vi "AWG IV measurement.vi"() -> ()   [LabVIEW 2024]
uses:
  <vilib>/LabVIEW Targets/FPGA/cRIO/shared/nicrio_ModuleControls/nicrio_cRIO-9775_TriggerSlope.ctl
  <vilib>/LabVIEW Targets/FPGA/cRIO/shared/nicrio_ModuleControls/nicrio_BasicConversionTime.ctl
  <vilib>/LabVIEW Targets/FPGA/cRIO/shared/nicrio_ModuleControls/nicrio_cRIO-9775_RecordDataRates4ChansRing.ctl
  Ramps.ctl
  <vilib>/rvi/Emulation/niFpgaGetClockAttributes.vi
  <vilib>/rvi/Emulation/niFpgaSctlEmulationGetInTimedLoop.vi
  <vilib>/rvi/Emulation/niFpgaEmulationReportErrorSimple.vi
  <vilib>/rvi/eio/common/nirviEmuTemplateMethod_errors.vi
  <vilib>/rvi/Emulation/niFpgaCriticalErrorInLSC.vi
  <vilib>/rvi/Emulation/niFpgaProcessEmulError.vi
  <vilib>/rvi/Emulation/niFpgaEmulationIsFPGAContextNoSignature.vi
  <vilib>/rvi/errors/niFpgaSetErrorForExecOnDevCompSimple.vi
  <vilib>/rvi/eio/common/nirviEmuReportErrorAndStop.vi
  <vilib>/rvi/DataTransferAndStorage/Container/Common/niFpgaContainerGetUniqueNameForEmu.vi
  <vilib>/rvi/FIFO/Fifo_Resource/nirvififoEmulationSetSize.vi
  <vilib>/rvi/FIFO/Fifo_Resource/nirviFifoEmulationQueueMgr.vi
  <instcachedir>/0/nirviFifoEmulationQueueMgr_E5CAEC123FF24DC58D834DCA3CDAA9B5.lvgen/nirviFifoEmulationQueueMgr_E5CAEC123FF24DC58D834DCA3CDAA9B5_001.vi
  <vilib>/rvi/FIFO/Fifo_Resource/nirvififoEmulationDetermineInputValidOut.vi
  <vilib>/rvi/FIFO/Fifo_Resource/nirvififoEmulationCreateLock.vi
  <vilib>/rvi/FIFO/Fifo_Resource/nirvififoEmulationObtainLock.vi
  <vilib>/rvi/FIFO/Fifo_Resource/nirvififoEmulationReleaseLock.vi
  <vilib>/rvi/occurrence/nirviWaitOnOccurrenceBase.vi
  <vilib>/rvi/errors/nirviReportUnexpectedCaseInternalError.vi
  <vilib>/rvi/errors/nirviReportUnexpectedCaseInternalError (U32).vi
  <vilib>/rvi/eio/common/nirviEmuTemplatePropertySet_errors.vi
  <vilib>/Utility/error.llb/Clear Errors.vi
  <vilib>/rvi/Memory/Memory_Emulation/nirvimemoryEmulation.vi
  <vilib>/rvi/Memory/Memory_Emulation/nirvimemoryFastEmulation.vi
  <vilib>/rvi/Memory/Memory_Emulation/niFpgaMemoryEmulationCacheClearOnFirstRun.vi
  <vilib>/rvi/Memory/Memory_Emulation/nirvimemoryEmulationManagerCache_MakeExclusive.vi
  <vilib>/rvi/Memory/Memory_Emulation/niFpgaMemoryEmulationValidateCache.vi
  <vilib>/rvi/Memory/Memory_Emulation/nirvimemoryEmulationManagerCache_InsertValue.vi
  <vilib>/rvi/Memory/Memory_Emulation/nirvimemoryEmulationManagerCache_ReleaseExclusive.vi
  <vilib>/rvi/Memory/Memory_Emulation/nirvimemoryEmulationManagerCache_GetValue.vi
  <vilib>/rvi/Memory/Memory_Emulation/nirvimemoryEmulationManagerCache_SetValue.vi
  <vilib>/rvi/Emulation/niFpgaSctlEmulationResourceMgr.vi
  <vilib>/eio/utilities/niEioResolveVilibRelativePath.vi
  <vilib>/rvi/interface/RandomDataEmulation/niFpgaRandomDataHandleErrors.vi
  <vilib>/rvi/DataTransferAndStorage/Container/Common/niFpgaContainerSetEmuInfo.vi
  <vilib>/eio/EIONode/EIONode.xnode
  <vilib>/rvi/DataTransferAndStorage/Container/XNode/niFpgaContainer.xnode
  <vilib>/rvi/FIFO/Fifo_Resource/nirvififoEmulationWrite.vi
  <vilib>/eio/EIOPropertyNode/EIOPropertyNode.xnode
  <vilib>/rvi/FIFO/Fifo_Resource/nirvififoEmulationRead.vi
  <vilib>/eio/EIOMethodNode/EIOMethodNode.xnode
  <vilib>/rvi/interface/RandomDataEmulation/nirviRandomDataFpgaReadWriteTemplate.vi
  <vilib>/rvi/LocalResourceManager/LocalResourceManager.xnode
  <vilib>/rvi/eio/common/nirviEmuTemplatePropertyGet_errors.vi
  <vilib>/rvi/eio/common/nirviEmuTemplatePropertyGet_noerrors.vi
  <vilib>/rvi/eio/common/nirviEmuTemplatePropertySet_noerrors.vi
panel:
  in  "Init gate":bool
  out "AWG pointer":u32
  in  "Ramps":T1={"Amp"=0.0, "Delay time 10us"=1, "Ramp1 time 10us"=1000, "Ramp2 time 10us"=2000, "Ramp3 time 10us"=1000, "End time 10us"=1}
  out "AWG length":u32
  in  "Trigger length ticks":u32=2 caption="Pulse ticks"
  in  "Cutoff delay usec":u32
  in  "Wait before trigger us":u32
  in  "Ic Cut off or curve":bool
  in  "Timeout":i32=-1
  in  "Record Samples":u32=25
  in  "Record PreTrigger Samples":u32=1
  in  "Record Data Rate":T2=1 items=["20.000 MS/s (NI 9775)"=1, "10.00 MS/s (NI 9775)"=2, "6.667 MS/s (NI 9775)"=3, "5.000 MS/s (NI 9775)"=4, "2.500 MS/s (NI 9775)"=8, "1.667 MS/s (NI 9775)"=12, "1.250 MS/s (NI 9775)"=16, "1.000 MS/s (NI 9775)"=20, "833.333 KS/s (NI 9775)"=24, "714.286 KS/s (NI 9775)"=28, "625.000 KS/s (NI 9775)"=32, "555.556 KS/s (NI 9775)"=36, "500.000 KS/s (NI 9775)"=40, "454.545 KS/s (NI 9775)"=44, "416.667 KS/s (NI 9775)"=48, "384.615 KS/s (NI 9775)"=52, "357.143 KS/s (NI 9775)"=56, "333.333 KS/s (NI 9775)"=60, "312.500 KS/s (NI 9775)"=64, "294.118 KS/s (NI 9775)"=68, "277.778 KS/s (NI 9775)"=72, "263.158 KS/s (NI 9775)"=76, "250.000 KS/s (NI 9775)"=80, "238.095 KS/s (NI 9775)"=84, "227.273 KS/s (NI 9775)"=88, "217.391 KS/s (NI 9775)"=92, "208.333 KS/s (NI 9775)"=96, "200.000 KS/s (NI 9775)"=100, "192.308 KS/s (NI 9775)"=104, "185.185 KS/s (NI 9775)"=108, "178.571 KS/s (NI 9775)"=112, "172.414 KS/s (NI 9775)"=116, "166.667 KS/s (NI 9775)"=120, "161.290 KS/s (NI 9775)"=124, "156.250 KS/s (NI 9775)"=128, "151.515 KS/s (NI 9775)"=132, "147.059 KS/s (NI 9775)"=136, "142.857 KS/s (NI 9775)"=140, "138.889 KS/s (NI 9775)"=144, "135.135 KS/s (NI 9775)"=148, "131.579 KS/s (NI 9775)"=152, "128.205 KS/s (NI 9775)"=156, "125.000 KS/s (NI 9775)"=160, "121.951 KS/s (NI 9775)"=164, "119.048 KS/s (NI 9775)"=168, "116.279 KS/s (NI 9775)"=172, "113.636 KS/s (NI 9775)"=176, "111.111 KS/s (NI 9775)"=180, "108.696 KS/s (NI 9775)"=184, "106.383 KS/s (NI 9775)"=188, "104.167 KS/s (NI 9775)"=192, "102.041 KS/s (NI 9775)"=196, "100.000 KS/s (NI 9775)"=200, "50.000 KS/s (NI 9775)"=400, "33.333 KS/s (NI 9775)"=600, "25.000 KS/s (NI 9775)"=800, "20.000 KS/s (NI 9775)"=1000, "16.667 KS/s (NI 9775)"=1200, "14.286 KS/s (NI 9775)"=1400, "12.500 KS/s (NI 9775)"=1600, "11.111 KS/s (NI 9775)"=1800, "10.000 KS/s (NI 9775)"=2000, "9.091 KS/s (NI 9775)"=2200, "8.333 KS/s (NI 9775)"=2400, "7.692 KS/s (NI 9775)"=2600, "7.143 KS/s (NI 9775)"=2800, "6.667 KS/s (NI 9775)"=3000, "6.250 KS/s (NI 9775)"=3200, "5.882 KS/s (NI 9775)"=3400, "5.556 KS/s (NI 9775)"=3600, "5.000 KS/s (NI 9775)"=4000, "4.762 KS/s (NI 9775)"=4200, "4.545 KS/s (NI 9775)"=4400, "4.348 KS/s (NI 9775)"=4600, "4.167 KS/s (NI 9775)"=4800, "4.000 KS/s (NI 9775)"=5000, "3.846 KS/s (NI 9775)"=5200, "3.571 KS/s (NI 9775)"=5600, "3.333 KS/s (NI 9775)"=6000, "3.125 KS/s (NI 9775)"=6400, "2.941 KS/s (NI 9775)"=6800, "2.778 KS/s (NI 9775)"=7200, "2.632 KS/s (NI 9775)"=7600, "2.500 KS/s (NI 9775)"=8000, "2.381 KS/s (NI 9775)"=8400, "2.273 KS/s (NI 9775)"=8800, "2.174 KS/s (NI 9775)"=9200, "2.083 KS/s (NI 9775)"=9600, "2.000 KS/s (NI 9775)"=10000, "1.923 KS/s (NI 9775)"=10400, "1.852 KS/s (NI 9775)"=10800, "1.786 KS/s (NI 9775)"=11200, "1.724 KS/s (NI 9775)"=11600, "1.667 KS/s (NI 9775)"=12000, "1.613 KS/s (NI 9775)"=12400, "1.563 KS/s (NI 9775)"=12800, "1.515 KS/s (NI 9775)"=13200, "1.471 KS/s (NI 9775)"=13600, "1.429 KS/s (NI 9775)"=14000, "1.389 KS/s (NI 9775)"=14400, "1.351 KS/s (NI 9775)"=14800, "1.316 KS/s (NI 9775)"=15200, "1.282 KS/s (NI 9775)"=15600, "1.250 KS/s (NI 9775)"=16000, "1.220 KS/s (NI 9775)"=16400, "1.190 KS/s (NI 9775)"=16800, "1.163 KS/s (NI 9775)"=17200, "1.136 KS/s (NI 9775)"=17600, "1.111 KS/s (NI 9775)"=18000, "1.087 KS/s (NI 9775)"=18400, "1.064 KS/s (NI 9775)"=18800, "1.042 KS/s (NI 9775)"=19200, "1.020 KS/s (NI 9775)"=19600, "1.000 KS/s (NI 9775)"=20000, "0.980 KS/s (NI 9775)"=20400, "0.962 KS/s (NI 9775)"=20800, "0.943 KS/s (NI 9775)"=21200, "0.926 KS/s (NI 9775)"=21600, "0.909 KS/s (NI 9775)"=22000, "0.893 KS/s (NI 9775)"=22400, "0.877 KS/s (NI 9775)"=22800, "0.862 KS/s (NI 9775)"=23200, "0.847 KS/s (NI 9775)"=23600, "0.833 KS/s (NI 9775)"=24000, "0.820 KS/s (NI 9775)"=24400, "0.806 KS/s (NI 9775)"=24800, "0.794 KS/s (NI 9775)"=25200, "0.781 KS/s (NI 9775)"=25600, "0.694 KS/s (NI 9775)"=28800, "0.625 KS/s (NI 9775)"=32000, "0.568 KS/s (NI 9775)"=35200, "0.521 KS/s (NI 9775)"=38400, "0.446 KS/s (NI 9775)"=44800, "0.391 KS/s (NI 9775)"=51200, "0.347 KS/s (NI 9775)"=57600, "0.313 KS/s (NI 9775)"=64000]
  in  "Timing Mode":T3
  in  "Records Num":i32
  in  "AI Trigger Configuration":T5={"Trigger Slope"=enum."Positive", "Trigger Level"=1.199951171875, "Hystesis Value"=1.10009765625, "AI Channel"=0}
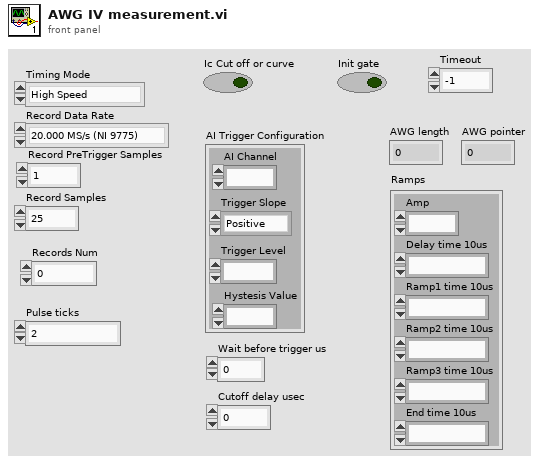
[diagram p1: front panel]
types:
  T1 = typedef "Ramps.ctl" = cluster{"Amp":fxp<+/-,20,5>, "Delay time 10us":i32, "Ramp1 time 10us":i32, "Ramp2 time 10us":i32, "Ramp3 time 10us":i32, "End time 10us":i32}
  T2 = typedef "nicrio_cRIO-9775_RecordDataRates4ChansRing.ctl" = u16
  T3 = typedef "nicrio_BasicConversionTime.ctl" = enum8{"High Speed", "High Resolution"}
  T4 = typedef "nicrio_cRIO-9775_TriggerSlope.ctl" = enum8{"Positive", "Negative"}
  T5 = cluster{"Trigger Slope":T4, "Trigger Level":fxp<+/-,17,5>, "Hystesis Value":fxp<+,16,4>, "AI Channel":u8}
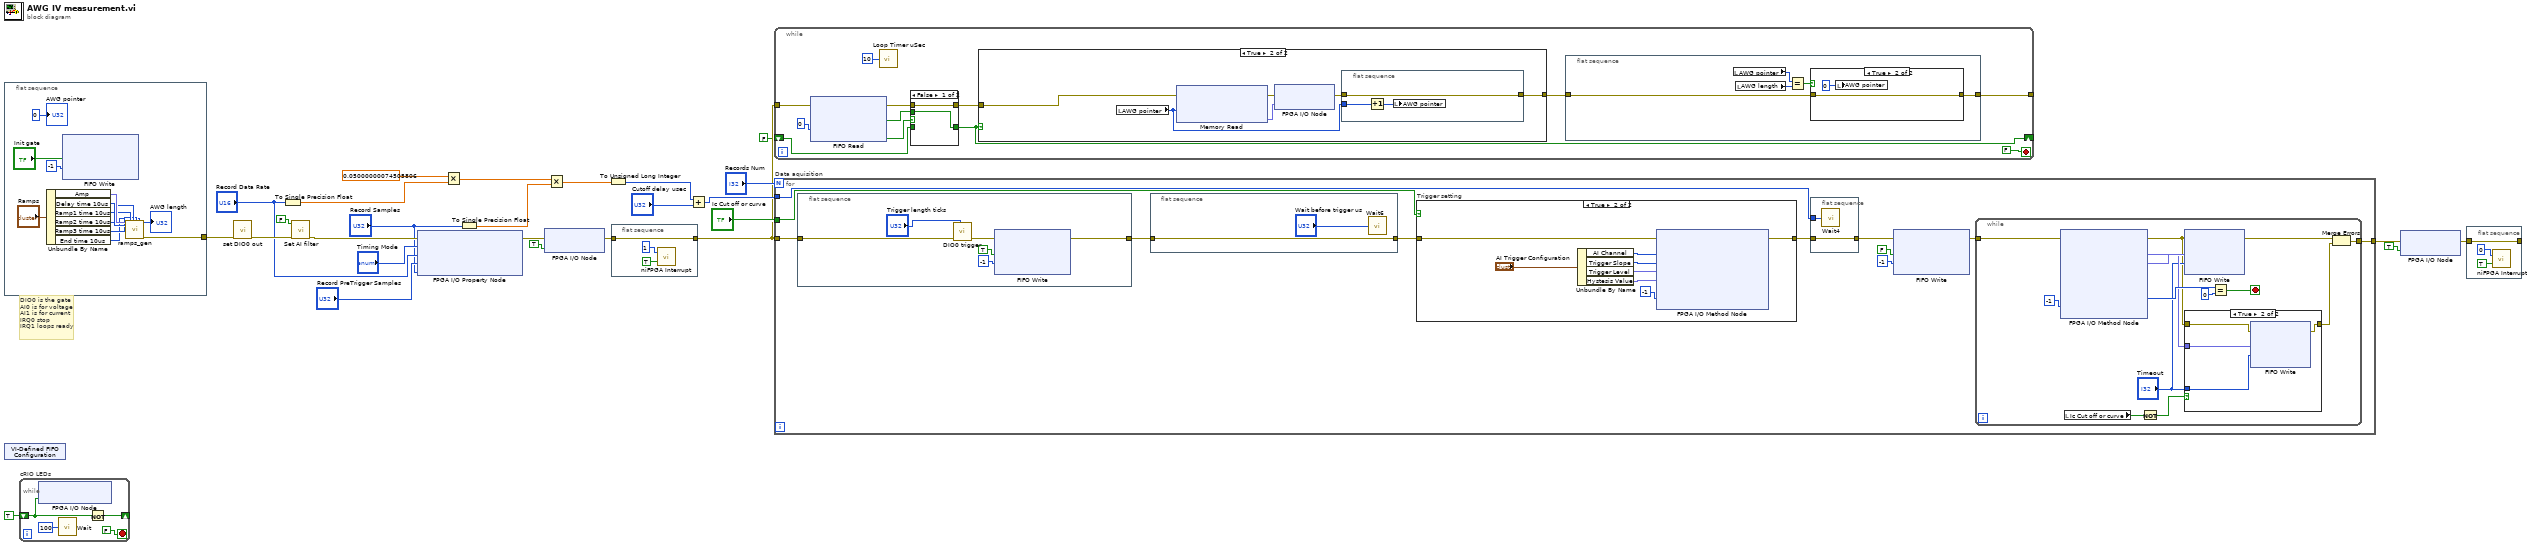
[diagram p0: block diagram]
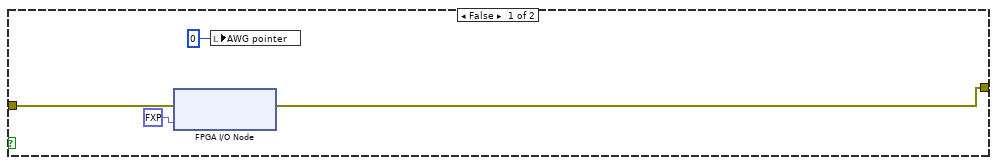
[diagram p4: hidden frame]
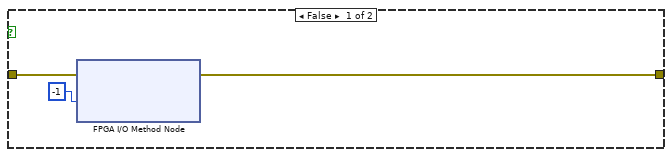
[diagram p5: hidden frame]
diagram:
  # "DIO0 is the gate\nAI0 is for voltage\nAI1 is for current\nIRQ0 stop\nIRQ1 loops ready"
  n1 = flat-sequence {
    tunnel: [w30] -> w5
    frame #0 {
      n2 = Unbundle By Name("Ramps") -> ("Amp"=w37:fxp<+/-,20,5>, "Delay time 10us"=w36:i32, "Ramp1 time 10us"=w35:i32, "Ramp2 time 10us"=w34:i32, "Ramp3 time 10us"=w33:i32, "End time 10us"=w32:i32)
      n3 = xnode ("FIFO Write")("Element"="Init gate", "Timeout"=-1) -> ()  [unwired: 1 in, 2 out]
      n4 = call "ramps_gen.vi"("Amp"=w37, "Delay time 10us"=w36, "Ramp1 time 10us"=w35, "Ramp2 time 10us"=w34, "Ramp3 time 10us"=w33, "End time 10us"=w32) -> ("End Address"=→"AWG length":u32, "error out"=w30:errorcluster)  [unwired: 12 in]
      "AWG pointer" <- u32 0 ("AWG pointer")
    }
  }
  n5 = xnode "VI-Defined FIFO Configuration"() -> ()  [unwired: 1 out]
  n6 = while "cRIO LEDs" {
    shift-right: [w41] -> _
    shift-left: TRUE ("USER FPGA LED") -> [w42]
    stop <- FALSE stop-if-true
    n7 = xnode "FPGA I/O Node"("USER FPGA LED"=w42) -> ()  [unwired: 1 in, 1 out]
    n8 = call "Wait"("Count(mSec)"=u32 100) -> ()  [unwired: 1 out]
    n9 = Not(x=w42) -> (.not. x?=w41:bool)
  }
  n10 = call "set DIO0 out.vi"("error in"=w5) -> ("error out"=w18:errorcluster)  [unwired: 10 in]
  n11 = To Single Precision Float(number="Record Data Rate") -> (single precision float=w13:sgl)
  n12 = call "Set AI filter.vi"("error in (no error)"=w18, "Enable All Low Pass Filter"=FALSE ("Enable Low Pass Filter")) -> ("error out"=w24:errorcluster)  [unwired: 9 in]
  n13 = xnode "FPGA I/O Property Node"("error in"=w24, "Timing Mode"="Timing Mode", "Record Data Rate"="Record Data Rate", "Record PreTrigger Samples"="Record PreTrigger Samples", "Record Samples"="Record Samples") -> ("error out"=w23:errorcluster)  [unwired: 1 in, 1 out]
  n14 = Multiply(x=sgl 0.05, y=w13) -> (x*y=w12:sgl)
  n15 = To Single Precision Float(number="Record Samples") -> (single precision float=w10:sgl)
  n16 = xnode "FPGA I/O Node"("error in"=w23, "Mod1/Start"=TRUE) -> ("error out"=w3:errorcluster)  [unwired: 1 in, 1 out]
  n17 = Multiply(x=w12, y=w10) -> (x*y=w9:sgl)
  n18 = To Unsigned Long Integer(number=w9) -> (unsigned 32bit integer=w8:u32)
  n19 = flat-sequence {
    tunnel: [w46] -> w2
    tunnel: w3 -> [w46]
    frame #0 {
      n20 = call <vilib>:"niFPGA Interrupt.vi"("Wait Until Cleared (F)"=TRUE, "IRQ Number (0)"=u8 1) -> ()  [unwired: 1 in]
    }
  }
  n21 = Add(x=w8, y="Cutoff delay usec") -> (x+y=w6:u32)
  n22 = while {
    tunnel: w2 -> [w49]
    tunnel: [w56] -> _
    shift-right: [w51] -> _
    shift-left: FALSE -> [w50]
    stop <- FALSE stop-if-true
    n23 = xnode ("FIFO Read")("Timeout"=0, "error in (no error)"=w49) -> ("Element"=w52:bool, "Timed Out?"=w53:bool, "error out"=w47:errorcluster)  [unwired: 1 in, 1 out]
    n24 = call "Loop Timer uSec"("Count(uSec)"=u32 10) -> ()  [unwired: 1 out]
    n25 = case shown="False" w53 {
      tunnel: [w60 w62] -> w51
      tunnel: w52 -> [w60 _]
      tunnel: w50 -> [_ w62]
      tunnel: [w59 w61] -> w48
      tunnel: w47 -> [w59 w61]
      frame False {
      }
      frame True {
      }
    }
    n26 = case shown="True" w51 {
      tunnel: w48 -> [w73 w80]
      tunnel: [w72 w76] -> w57
      frame False {
        n27 = xnode "FPGA I/O Node"("error in"=w73, "Mod3/AO0"=fxp<+/-,20,5> 0.0) -> ("error out"=w72:errorcluster)  [unwired: 1 in, 1 out]
        n28 = local write "AWG pointer"(u32 0 ("AWG pointer")) -> ()
      }
      frame True {
        n29 = local read "AWG pointer"() -> (w78:u32)
        n30 = xnode ("Memory Read")("Address"=w78, "error in (no error)"=w80) -> ("Data"=w75:fxp<+/-,20,5>, "error out"=w79:errorcluster)  [unwired: 1 in, 1 out]
        n31 = xnode "FPGA I/O Node"("error in"=w79, "Mod3/AO0"=w75) -> ("error out"=w77:errorcluster)  [unwired: 1 in, 1 out]
        n32 = flat-sequence {
          tunnel: w78 -> [w83]
          tunnel: [w81] -> w76
          tunnel: w77 -> [w81]
          frame #0 {
            n33 = Increment(x=w83) -> (x+1=w82:u32)
            n34 = local write "AWG pointer"(w82) -> ()
          }
        }
      }
    }
    n35 = flat-sequence {
      tunnel: w57 -> [w64]
      tunnel: [w63] -> w56
      frame #0 {
        n36 = local read "AWG pointer"() -> (w67:u32)
        n37 = local read "AWG length"() -> (w66:u32)
        n38 = Equal?(x=w67, y=w66) -> (x = y?=w65:bool)
        n39 = case shown="True" w65 {
          tunnel: w64 -> [w68 w69]
          tunnel: [w68 w69] -> w63
          frame False {
          }
          frame True {
            n40 = local write "AWG pointer"(u32 0 ("AWG pointer")) -> ()
          }
        }
      }
    }
  }
  n41 = for "Data aquisition" {
    N: "Records Num" -> [_]
    tunnel: w2 -> [w92]
    tunnel: "Ic Cut off or curve" -> [w93]
    tunnel: [w94] -> w17
    tunnel: w6 -> [w90]
    n42 = flat-sequence {
      tunnel: w92 -> [w103]
      tunnel: [w99] -> w85
      frame #0 {
        n43 = call "DIO0 trigger.vi"("Pulse ticks"="Trigger length ticks", "error in"=w103) -> ("error out"=w100:errorcluster)  [unwired: 9 in]
        n44 = xnode ("FIFO Write")("Element"=TRUE, "Timeout"=-1, "error in (no error)"=w100) -> ("error out"=w99:errorcluster)  [unwired: 1 in, 2 out]
      }
    }
    n45 = flat-sequence {
      tunnel: w85 -> [w95]
      tunnel: [w95] -> w84
      frame #0 {
        n46 = call "Wait6"("Count(uSec)"="Wait before trigger us") -> ()  [unwired: 1 out]
      }
    }
    n47 = case "Trigger setting" shown="True" w93 {
      tunnel: w84 -> [w106 w108]
      tunnel: [w105 w109] -> w91
      frame False {
        n48 = xnode "FPGA I/O Method Node"("error in"=w106, "Timeout (Ticks)"=-1) -> ("error out"=w105:errorcluster)  [unwired: 1 in, 2 out]
      }
      frame True {
        n49 = Unbundle By Name("AI Trigger Configuration") -> ("AI Channel"=w115:u8, "Trigger Slope"=w114:T4, "Trigger Level"=w113:fxp<+/-,17,5>, "Hystesis Value"=w112:fxp<+,16,4>)
        n50 = xnode "FPGA I/O Method Node"("error in"=w108, "AI Channel"=w115, "Trigger Slope"=w114, "Trigger Level"=w113, "Hysteresis Value"=w112, "Timeout (Ticks)"=-1) -> ("error out"=w109:errorcluster)  [unwired: 1 in, 3 out]
      }
    }
    n51 = flat-sequence {
      tunnel: w91 -> [w98]
      tunnel: w90 -> [w97]
      tunnel: [w98] -> w87
      frame #0 {
        n52 = call "Wait4"("Count(uSec)"=w97) -> ()  [unwired: 1 out]
      }
    }
    n53 = xnode ("FIFO Write")("Element"=FALSE, "Timeout"=-1, "error in (no error)"=w87) -> ("error out"=w86:errorcluster)  [unwired: 1 in, 2 out]
    n54 = while {
      tunnel: w86 -> [w129]
      tunnel: [w118] -> w94
      stop <- w125 stop-if-true
      n55 = xnode "FPGA I/O Method Node"("error in"=w129, "Timeout (Ticks)"=-1) -> ("error out"=w121:errorcluster, "AI0"=w123:fxp<+/-,17,5>, "AI1"=w124:fxp<+/-,17,5>, "Elements Remaining"=w127:u32)  [unwired: 1 in, 5 out]
      n56 = local read "Ic Cut off or curve"() -> (w117:bool)
      n57 = Not(x=w117) -> (.not. x?=w116:bool)
      n58 = xnode ("FIFO Write")("Element"=w124, "Timeout"="Timeout", "error in (no error)"=w121) -> ("error out"=w120:errorcluster)  [unwired: 1 in, 2 out]
      n59 = case shown="True" w116 {
        tunnel: w123 -> [_ w134]
        tunnel: "Timeout" -> [_ w133]
        tunnel: w121 -> [w130 w132]
        tunnel: [w130 w131] -> w119
        frame False {
        }
        frame True {
          n60 = xnode ("FIFO Write")("Element"=w134, "Timeout"=w133, "error in (no error)"=w132) -> ("error out"=w131:errorcluster)  [unwired: 1 in, 2 out]
        }
      }
      n61 = Equal?(x=w127, y=u32 0) -> (x = y?=w125:bool)
      n62 = Merge Errors(w120, w119) -> (w118:errorcluster)
    }
  }
  n63 = xnode "FPGA I/O Node"("error in"=w17, "Mod1/Stop"=TRUE) -> ("error out"=w16:errorcluster)  [unwired: 1 in, 1 out]
  n64 = flat-sequence {
    tunnel: w16 -> [w137]
    tunnel: [w137] -> _
    frame #0 {
      n65 = call <vilib>:"niFPGA Interrupt.vi"("Wait Until Cleared (F)"=TRUE, "IRQ Number (0)"=u8 0) -> ()  [unwired: 1 in]
    }
  }
